vi "setup.vi"(11 "PicamModel":T1=715 items=["---PIXIS 100 SERIES---"=1000, "PixisSeries"=0, "Pixis100BR"=5, "---PI-MAX4 SERIES---"=1001, "Pimax4Series"=700, "PiMax41024EM"=715]) -> (0 "error out":errorcluster, 3 "Picam out":refnum<class "Picam.lvclass">)   [LabVIEW 2019, in "Picam.lvclass"]
uses:
  Picam.lvclass
  picam32_LabView_SDK/PICam_lib/types/PicamModel.ctl
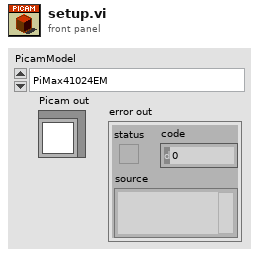
[diagram p1: front panel]
types:
  T1 = typedef "PicamModel.ctl" = u32
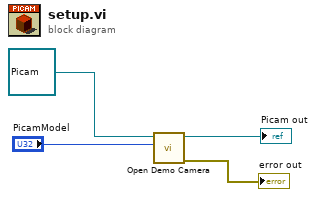
[diagram p0: block diagram]
diagram:
  n1 = call-dynamic "Open Demo Camera.vi"("PicamModel"="PicamModel", "Picam in"=refnum<class "Picam.lvclass"> refnum) -> ("error out"=→"error out":errorcluster, "Picam out"=→"Picam out":refnum<class "Picam.lvclass">)  [unwired: 8 in]
